vi "ElevatorSystemMoveElevatorToSetpoint.vi"(1 "Device Names":string[](array[string]), 2 "Scoring Heights":i32[](array[numeric]), 3 "Target Position":T2(ring)=enum."Low (Hooks rest under lip)") -> (0 "Elevator Status":T1)   [LabVIEW 2014]
panel:
  # "Scoring"
  # "Low"
  # "High"
  # "Proximity Sensor"
  # "Elevator Encoder"
  # "Elevator Motor"
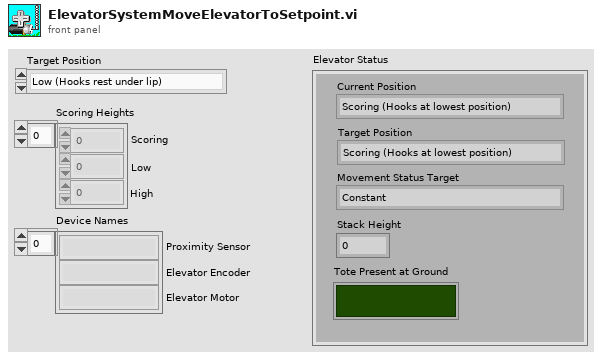
[diagram p1: front panel]
types:
  T1 = cluster{"Current Position":enum16{"Scoring (Hooks at lowest position)", "Intermediary (Between positions)", "Low (Hooks rest under lip)", "High (Holding totes up)"}, "Movement Status Target":enum16{"Constant", "Lifting", "Lowering"}, "Stack Height":i32, "Tote Present at Ground":bool, "Target Position":enum16{"Scoring (Hooks at lowest position)", "Low (Hooks rest under lip)", "High (Holding totes up)", "Intermediary"}}
  T2 = enum16{"Scoring (Hooks at lowest position)", "Low (Hooks rest under lip)", "High (Holding totes up)"}
  T3 = cluster{"Current Position":enum16{"Scoring (Hooks at lowest position)", "Intermediary (Between positions)", "Low (Hooks rest under lip)", "High (Holding totes up)"}, "Movement Status Target":enum16{"Constant", "Lifting", "Lowering"}, "Stack Height":i32, "Tote Present at Ground":bool, "Target Position":enum16{"Scoring (Hooks at lowest position)", "Low (Hooks rest under lip)", "High (Holding totes up)"}}
  T4 = typedef "WPI_DigitalInputDevRef.ctl" = cluster{"DevStatus":errorcluster, "DIO Channel":T5, "Controller":T6}
  T5 = typedef "FPGA_DIOChannel.ctl" = enum8{"DIO 0", "DIO 1", "DIO 2", "DIO 3", "DIO 4", "DIO 5", "DIO 6", "DIO 7", "DIO 8", "DIO 9", "DIO MXP 0", "DIO MXP 1", "DIO MXP 2", "DIO MXP 3", "DIO MXP 4", "DIO MXP 5", "DIO MXP 6", "DIO MXP 7", "DIO MXP 8", "DIO MXP 9", "DIO MXP 10", "DIO MXP 11", "DIO MXP 12", "DIO MXP 13", "DIO MXP 14", "DIO MXP 15", "Invalid"}
  T6 = typedef "FPGA_TypedefDigitalModule.ctl" = enum16{"Controller 1"}
  T7 = typedef "WPI_EncoderDevRef.ctl" = cluster{"DevStatus":errorcluster, "EncoderIndex":T8, "CounterIndex":T9, "DistancePerCount":dbl, "Decoding Type":T10}
  T8 = typedef "FPGA_EncoderIdx.ctl" = enum8{"Enc 0", "Enc 1", "Enc 2", "Enc 3", "Enc 4", "Enc 5", "Enc 6", "Enc 7", "Invalid"}
  T9 = typedef "FPGA_CounterCtrSystemIndex.ctl" = enum8{"Ctr 0", "Ctr 1", "Ctr 2", "Ctr 3", "Ctr 4", "Ctr 5", "Ctr 6", "Ctr 7", "Invalid"}
  T10 = typedef "WPI_EncoderType.ctl" = enum16{"1x", "2x", "4x"}
  T11 = typedef "WPI_MotorControlDeviceRef.ctl" = cluster{"DeviceStatus":errorcluster, "Type":T12, "PWM":cluster{"Controller":T6, "PWM Channel":T13, "DeadBand":T14}, "CAN":cluster{"Device Number":u8, "Control Mode":T15, "Semaphore":T16, "Max Vout":dbl, "TalonSRX Control Mode":T17}, "Invert":bool, "TransformRef":T18, "InvTransformRef":T18}
  T12 = typedef "WPI_MotorControlType.ctl" = enum16{"PWM", "CAN", "CANTalonSRX"}
  T13 = typedef "FPGA_DIOPWMChannel.ctl" = enum8{"PWM 0", "PWM 1", "PWM 2", "PWM 3", "PWM 4", "PWM 5", "PWM 6", "PWM 7", "PWM 8", "PWM 9", "PWM MXP 0", "PWM MXP 1", "PWM MXP 2", "PWM MXP 3", "PWM MXP 4", "PWM MXP 5", "PWM MXP 6", "PWM MXP 7", "PWM MXP 8", "PWM MXP 9", "Invalid"}
  T14 = typedef "WPI_PWMDeadband.ctl" = cluster{"Name":string, "maxPositivePwm":i32, "minPositivePwm":i32, "centerPwm":i32, "maxNegativePwm":i32, "minNegativePwm":i32, "angularRange":u16}
  T15 = typedef "WPI_CANJaguar_ControlMode.ctl" = enum8{"Percent VBus", "Current", "Speed", "Position", "Voltage"}
  T16 = typedef "Semaphore RefNum" = refnum<k1>
  T17 = typedef "WPI_CANTalonSRX_APIControlMode.ctl" = enum8{"Percent VBus", "Speed", "Position", "Slave", "Unchanged / Invalid"}
  T18 = typedef "WPI_PWMTransform_ConPane.ctl" = refnum<vi>
  T19 = enum16{"Scoring (Hooks at lowest position)", "Intermediary (Between positions)", "Low (Hooks rest under lip)", "High (Holding totes up)"}
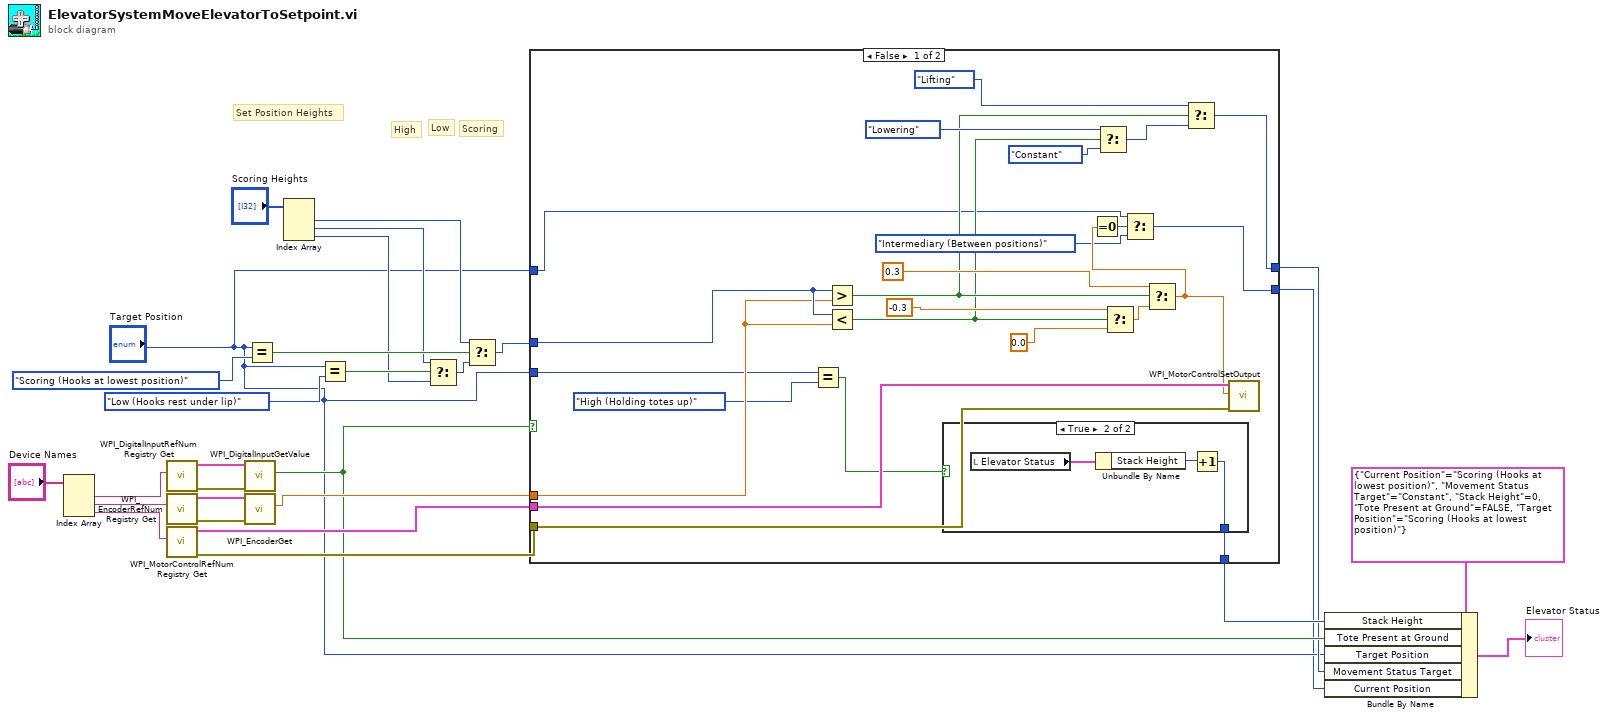
[diagram p0: block diagram]
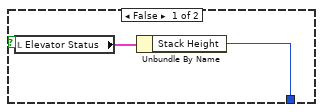
[diagram p2: hidden frame]
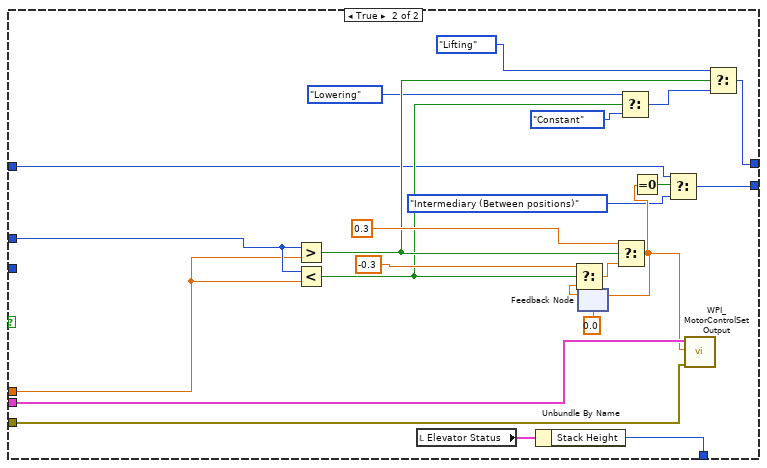
[diagram p3: hidden frame]
diagram:
  # "Scoring"
  # "Low"
  # "High"
  # "Set Position Heights"
  n1 = Index Array(array="Device Names") -> (element #1=w18:string, element #2=w17:string, element #3=w16:string)  [unwired: 3 in]
  n2 = call <vilib>:"WPI_DigitalInputRefNum Registry Get.vi"("refnum name"=w18) -> ("error out"=w15:errorcluster, "DigitalInputDevRef"=w14:T4)  [unwired: 9 in]
  n3 = call <vilib>:"WPI_EncoderRefNum Registry Get.vi"("refnum name"=w17) -> ("error out"=w13:errorcluster, "EncoderDevRef"=w12:T7)  [unwired: 9 in]
  n4 = call <vilib>:"WPI_MotorControlRefNum Registry Get.vi"("refnum name"=w16) -> ("error out"=w9:errorcluster, "MotorControlDevRef"=w10:T11)  [unwired: 9 in]
  n5 = call <vilib>:"WPI_DigitalInputGetValue.vi"("error in (no error)"=w15, "DigitalInputDevRef"=w14) -> ("Value"=w4:bool)  [unwired: 7 in, 2 out]
  n6 = call <vilib>:"WPI_EncoderGet.vi"("error in (no error)"=w13, "EncoderDevRef"=w12) -> ("Distance"=w11:dbl)  [unwired: 4 in, 5 out]
  n7 = Equal?(x="Target Position", y=T2."Scoring (Hooks at lowest position)") -> (x = y?=w27:bool)
  n8 = Index Array(array="Scoring Heights") -> (element #1=w25:i32, element #2=w21:i32, element #3=w20:i32)  [unwired: 3 in]
  n9 = Equal?(x="Target Position", y=T2."Low (Hooks rest under lip)") -> (x = y?=w23:bool)
  n10 = Select(t=w21, s=w23, f=w20) -> (s? t:f=w24:i32)
  n11 = Select(t=w25, s=w27, f=w24) -> (s? t:f=w8:i32)
  n12 = case shown="False" w4 {
    tunnel: w11 -> [w46 w79]
    tunnel: w10 -> [w52 w75]
    tunnel: w9 -> [w51 w74]
    tunnel: w8 -> [w47 w80]
    tunnel: [w44 w70] -> w5
    tunnel: "Target Position" -> [w43 _]
    tunnel: [w34 w68] -> w3
    tunnel: "Target Position" -> [w29 w60]
    tunnel: [w33 w58] -> w1
    frame False {
      n13 = Equal?(x=w43, y=T2."High (Holding totes up)") -> (x = y?=w41:bool)
      n14 = Greater?(x=w47, y=w46) -> (0:w36:bool)
      n15 = Less?(x=w47, y=w46) -> (x < y?=w35:bool)
      n16 = case shown="True" w41 {
        tunnel: [w53 w55] -> w44
        frame False {
          n17 = local read "Elevator Status"() -> (w54:T1)
          n18 = Unbundle By Name(w54) -> ("Stack Height"=w53:i32)
        }
        frame True {
          n19 = local read "Elevator Status"() -> (w57:T1)
          n20 = Unbundle By Name(w57) -> ("Stack Height"=w56:i32)
          n21 = Increment(x=w56) -> (x+1=w55:i32)
        }
      }
      n22 = Select(t=enum16{"Constant", "Lifting", "Lowering"}."Lowering" ("Movement Status Target"), s=w35, f=enum16{"Constant", "Lifting", "Lowering"}."Constant" ("Movement Status Target")) -> (s? t:f=w39:enum16{"Constant", "Lifting", "Lowering"})
      n23 = Select(t=-0.3, s=w35, f=0.0 ("t")) -> (s? t:f=w49:dbl)
      n24 = Select(t=0.3, s=w36, f=w49) -> (s? t:f=w31:dbl)
      n25 = Equal To 0?(x=w31) -> (x = 0?=w32:bool)
      n26 = Select(t=w29, s=w32, f=T19."Intermediary (Between positions)" ("Current Position")) -> (s? t:f=w33:u16)
      n27 = Select(t=enum16{"Constant", "Lifting", "Lowering"}."Lifting" ("Movement Status Target"), s=w36, f=w39) -> (s? t:f=w34:enum16{"Constant", "Lifting", "Lowering"})
      n28 = call <vilib>:"WPI_MotorControlSetOutput.vi"("error in (no error)"=w51, "Output"=w31, "MotorControlDevRef"=w52) -> ()  [unwired: 6 in, 3 out]
    }
    frame True {
      n29 = Greater?(x=w80, y=w79) -> (0:w69:bool)
      n30 = Less?(x=w80, y=w79) -> (x < y?=w65:bool)
      n31 = local read "Elevator Status"() -> (w71:T1)
      n32 = Unbundle By Name(w71) -> ("Stack Height"=w70:i32)
      n33 = feedback #1(0.0 ("t")) -> (w73:dbl)
      n34 = Select(t=-0.3, s=w65, f=w73) -> (s? t:f=w77:dbl)
      n35 = Select(t=0.3, s=w69, f=w77) -> (s? t:f=w61:dbl)
      n36 = feedback-in #1(w61) -> ()
      n37 = Select(t=enum16{"Constant", "Lifting", "Lowering"}."Lowering" ("Movement Status Target"), s=w65, f=enum16{"Constant", "Lifting", "Lowering"}."Constant" ("Movement Status Target")) -> (s? t:f=w66:enum16{"Constant", "Lifting", "Lowering"})
      n38 = Equal To 0?(x=w61) -> (x = 0?=w62:bool)
      n39 = Select(t=w60, s=w62, f=T19."Intermediary (Between positions)" ("Current Position")) -> (s? t:f=w58:u16)
      n40 = call <vilib>:"WPI_MotorControlSetOutput.vi"("error in (no error)"=w74, "Output"=w61, "MotorControlDevRef"=w75) -> ()  [unwired: 6 in, 3 out]
      n41 = Select(t=enum16{"Constant", "Lifting", "Lowering"}."Lifting" ("Movement Status Target"), s=w69, f=w66) -> (s? t:f=w68:enum16{"Constant", "Lifting", "Lowering"})
    }
  }
  n42 = Bundle By Name(cluster=T3 {"Current Position"=enum."Scoring (Hooks at lowest position)", "Movement Status Target"=enum."Constant", "Stack Height"=0, "Tote Present at Ground"=FALSE, "Target Position"=enum."Scoring (Hooks at lowest position)"} ("Elevator Status 2"), "Stack Height"=w5, "Tote Present at Ground"=w4, "Target Position"="Target Position", "Movement Status Target"=w3, "Current Position"=w1) -> (→"Elevator Status":T3)
